vi "MatchRegExJitToSubstringOffsets.vi"(5 "MatchOptions":u32 format="%.0x", 7 "CompileOptions":u32 format="%.0x", 8 "error in":errorcluster, 9 "offset (0)":i32, 10 "search pattern":string, 11 "string":string) -> (0 "error out":errorcluster, 1 "NoMatch?":bool, 2 "OffsetsPastMatch":i32[](array[numeric]), 3 "MatchOffsets":i32[](array[numeric]))   [LabVIEW 2021, in "libpcre2-8.lvlib"]
uses:
  libpcre2-8.lvlib
  Pcre2GetOvectorPointer8.vi
  Pcre2CompileError.vi
  Pcre2FnkCallError.vi
  Pcre2ErrorNull.vi
  Pcre2LibError.vi
panel:
  in  "JitOptions":u32=1 format="%.0x"
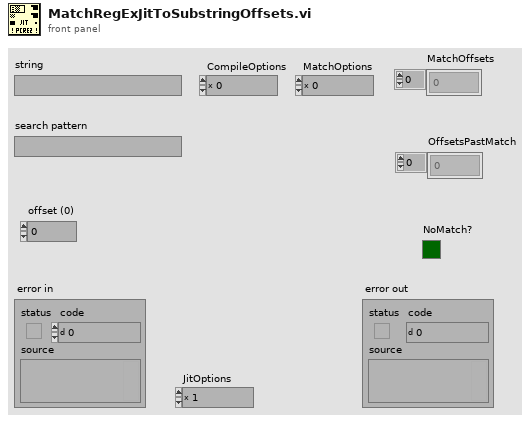
[diagram p1: front panel]
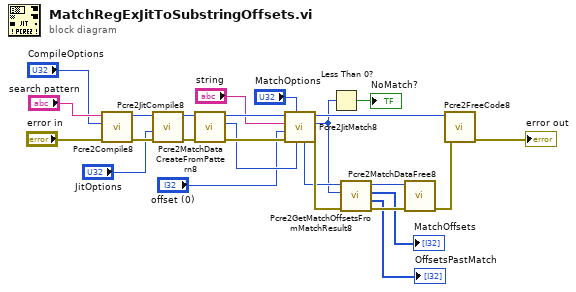
[diagram p0: block diagram]
diagram:
  n1 = call "Pcre2Compile8.vi"("error in"="error in", "Options"="CompileOptions", "Pattern"="search pattern") -> ("error out"=w7:errorcluster, "pCode"=w6:u64)  [unwired: 7 in]
  n2 = call "Pcre2JitCompile8.vi"("error in"=w7, "Options (1)"="JitOptions", "pCode"=w6) -> ("error out"=w8:errorcluster, "pCode"=w9:u64)  [unwired: 7 in]
  n3 = call "Pcre2MatchDataCreateFromPattern8.vi"("error in"=w8, "pCode"=w9) -> ("error out"=w24:errorcluster, "pMatchData"=w23:u64, "pCode"=w25:u64)  [unwired: 7 in]
  n4 = call "Pcre2JitMatch8.vi"("pMatchData"=w23, "Options"="MatchOptions", "error in"=w24, "StartOffset"="offset (0)", "Subject"="string", "pCode"=w25) -> ("error out"=w11:errorcluster, "MatchResult"=w2:i32, "pCode"=w22:u64, "pMatchData"=w10:u64)  [unwired: 2 in]
  n5 = Less Than 0?(x=w2) -> (x < 0?=→"NoMatch?":bool)
  n6 = call "Pcre2GetMatchOffsetsFromMatchResult8.vi"("error in"=w11, "MatchResult"=w2, "pMatchData"=w10) -> ("error out"=w17:errorcluster, "OffsetsPastMatch"=→"OffsetsPastMatch":i32[], "MatchOffsets"=→"MatchOffsets":i32[], "pMatchData"=w16:u64)  [unwired: 5 in]
  n7 = call "Pcre2MatchDataFree8.vi"("error in"=w17, "pMatchData"=w16) -> ("error out"=w21:errorcluster)  [unwired: 9 in]
  n8 = call "Pcre2FreeCode8.vi"("error in"=w21, "pCode"=w22) -> ("error out"=→"error out":errorcluster)  [unwired: 9 in]
